vi "subvi_Variant to String Array.vi"(10 "File Type":string, 11 "Variant":variant) -> (2 "File Information":string[][](array[string]), 3 "Header":string[](array[string]))   [LabVIEW 2016]
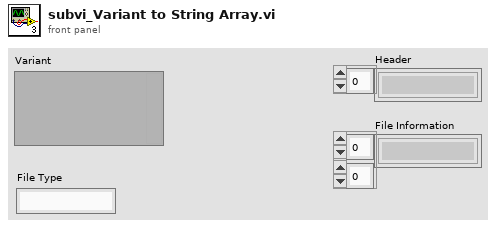
[diagram p1: front panel]
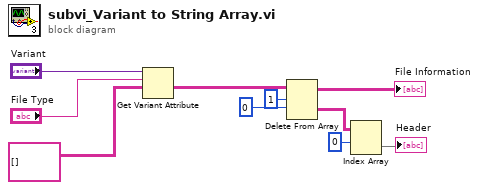
[diagram p0: block diagram]
diagram:
  n1 = Get Variant Attribute(Variant="Variant", name="File Type", default value (empty Variant)=string[][] []) -> (value=w7:string[][])  [unwired: 1 in, 3 out]
  n2 = Delete From Array(array=w7, length=1, index (row)=0) -> (deleted portion=w3:string[][], array with subset deleted=→"File Information":string[][])  [unwired: 1 in]
  n3 = Index Array(array=w3, index (row)=0) -> (element=→"Header":string[])  [unwired: 1 in]
